vi "Example.vi"() -> ()   [LabVIEW 2011]
doc: "This example shows how to use the Uniblitz driver for LabVIEW provided by Sixclear."
uses:
  driver/UNIBLITZ-Operation.ctl
  driver/UNIBLITZ-Address.ctl
  driver/UNIBLITZ-SteadyState.ctl
panel:
  in  "Simulation Mode?":bool
  in  "Send":bool
  in  "Steady State":T1
  in  "Address":T2
  in  "Uniblitz Shutter Operation":T3
  in  "VISA resource name":refnum<visa-resource-name>="COM1"
  out "error out":errorcluster
  in  "stop":bool
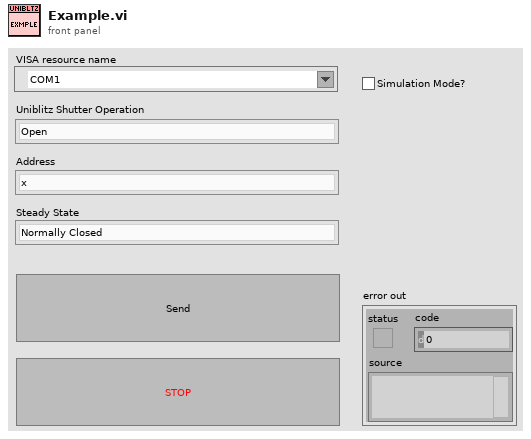
[diagram p1: front panel]
types:
  T1 = typedef "UNIBLITZ-SteadyState.ctl" = enum16{"Normally Closed", "Normally Open"}
  T2 = typedef "UNIBLITZ-Address.ctl" = enum16{"x", "0", "1", "2", "3", "4", "5", "6", "7"}
  T3 = typedef "UNIBLITZ-Operation.ctl" = enum8{"Open", "Close", "Trigger", "Reset", "AUX Enable", "AUX Disable", "Gate On", "Gate Off"}
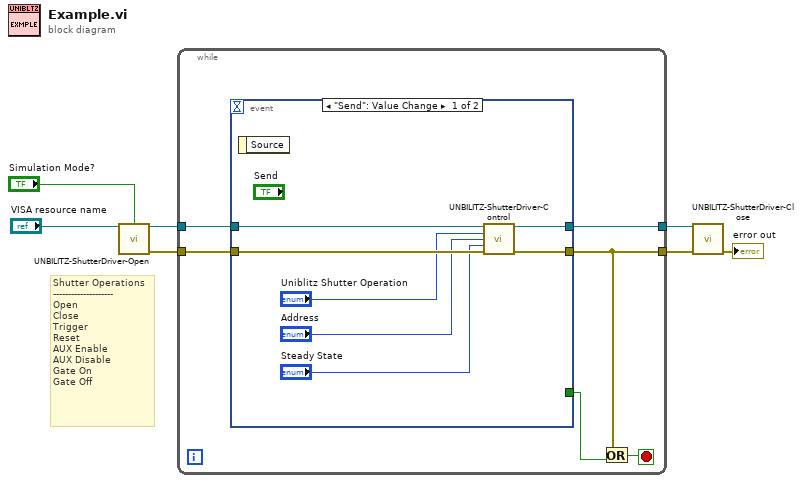
[diagram p0: block diagram]
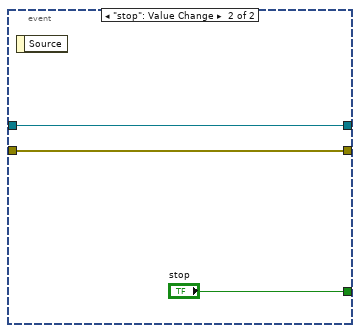
[diagram p2: hidden frame]
diagram:
  # "Shutter Operations\n--------------------\nOpen\nClose\nTrigger\nReset\nAUX Enable\nAUX Disable\nGate On\nGate Off"
  n1 = call "UNBILITZ-ShutterDriver-Open.vi"("VISA resource name"="VISA resource name", "Simulation Mode?"="Simulation Mode?") -> ("VISA resource name out"=w7:refnum<visa-resource-name>, "error out"=w6:errorcluster)  [unwired: 12 in]
  n2 = while {
    tunnel: w7 -> [w13]
    tunnel: w6 -> [w12]
    tunnel: [w11] -> w5
    tunnel: [w8] -> w4
    stop <- w10 stop-if-true
    n3 = event shown="[0] \"Send\": Value Change" {
      selector: _ -> [_ _]
      dyn-events: _ -> [_ _]
      timeout: _ -> [_ _]
      tunnel: w13 -> [w20 w22]
      tunnel: w12 -> [w19 w21]
      tunnel: [w18 w22] -> w11
      tunnel: [w17 w21] -> w8
      tunnel: [_ "stop"] -> w9
      event "Send": Value Change {
        n4 = event-data() -> ()  [unwired: 1 in, 1 out]
        n5 = call "UNBILITZ-ShutterDriver-Control.vi"("VISA resource name"=w20, "Uniblitz Operation"="Uniblitz Shutter Operation", "Address"="Address", "Steady State"="Steady State", "error in (no error)"=w19) -> ("VISA resource name out"=w18:refnum<visa-resource-name>, "error out"=w17:errorcluster)  [unwired: 9 in]
      }
      event "stop": Value Change {
        n6 = event-data() -> ()  [unwired: 1 in, 1 out]
      }
    }
    n7 = Or(x=w8, y=w9) -> (x .or. y?=w10:bool)
  }
  n8 = call "UNBILITZ-ShutterDriver-Close.vi"("VISA resource name"=w5, "error in (no error)"=w4) -> ("error out"=→"error out":errorcluster)  [unwired: 13 in]
